vi "create_txtfile.vi"(0 "appended path":path, 1 "append to file? (new file:F)":bool=TRUE, 2 "alternate path":path, 3 "String":string, 4 "String 2":string, 5 "String 3":string, 6 "String 6":string, 7 "String 4":string, 8 "String 12":string, 9 "String 14":string, 10 "String 13":string, 11 "String 15":string, 12 "String 5":string, 13 "String 9":string, 14 "String 7":string, 15 "String 8":string, 16 "Save in second location?":bool, 17 "String 10":string, 18 "String 11":string) -> (19 "concatenated string":string)   [LabVIEW 2013]
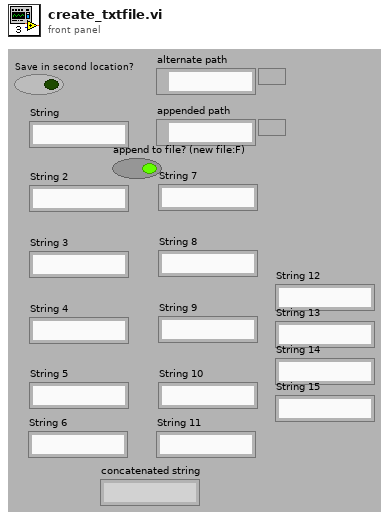
[diagram p1: front panel]
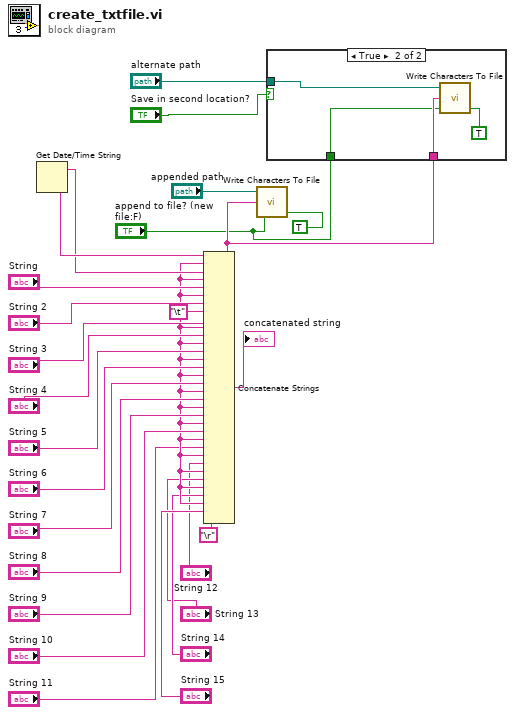
[diagram p0: block diagram]
diagram:
  w10 = "\t"
  n1 = Get Date/Time String() -> (date string=w18:string, time string=w19:string)  [unwired: 3 in]
  n2 = Concatenate Strings(w19, w10, w18, w10, "String", w10, "String 2", w10, "String 3", w10, "String 4", w10, "String 5", w10, "String 6", w10, "String 7", w10, "String 8", w10, "String 9", w10, "String 10", w10, "String 11", w10, "String 12", w10, "String 13", w10, "String 14", w10, "String 15", "\r") -> (w2:string)
  "concatenated string" <- w2
  n3 = call <vilib>:"Write Characters To File.vi"("convert eol? (no:F)"=TRUE, "append to file? (new file:F)"="append to file? (new file:F)", "character string"=w2, "file path (dialog if empty)"="appended path") -> ()  [unwired: 1 in, 1 out]
  n4 = case shown="True" "Save in second location?" {
    tunnel: "alternate path" -> [_ w28]
    tunnel: w2 -> [_ w27]
    tunnel: "append to file? (new file:F)" -> [_ w26]
    frame False {
    }
    frame True {
      n5 = call <vilib>:"Write Characters To File.vi"("convert eol? (no:F)"=TRUE, "append to file? (new file:F)"=w26, "character string"=w27, "file path (dialog if empty)"=w28) -> ()  [unwired: 1 in, 1 out]
    }
  }
